vi "radio_set_generate_msg.vi"(8 "error in":errorcluster, 9 "Radio command":u16(ring) items=["op mode", "frequency", "power", "spread factor", "freq correction", "RX signal bw", "bitrate", "freq deviation", "preamble length", "crc", "bandwidth"], 10 "input parameter":string, 11 "VISA in":refnum<visa-resource-name>) -> (0 "error out":errorcluster, 1 "error":bool, 2 "output command":string, 3 "VISA out":refnum<visa-resource-name>)   [LabVIEW 2011]
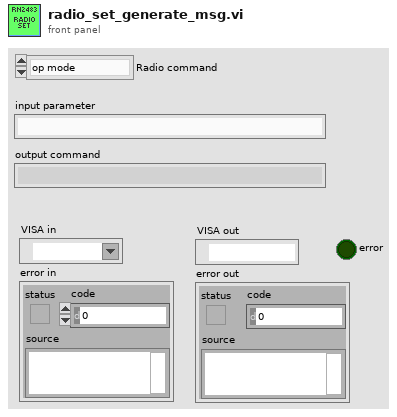
[diagram p1: front panel]
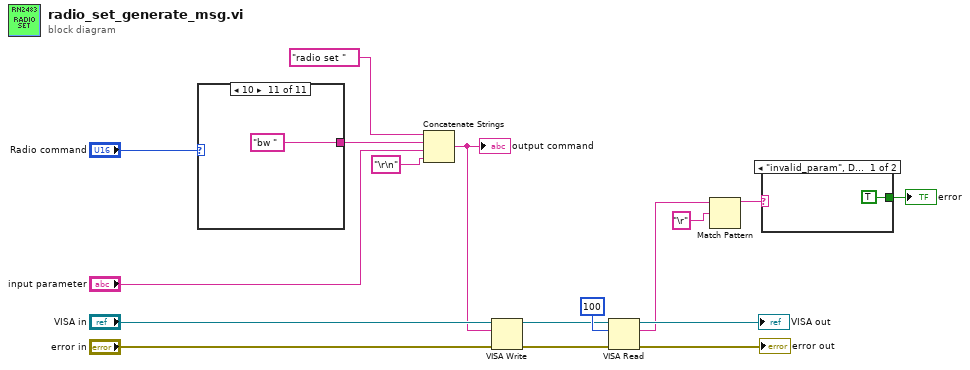
[diagram p0: block diagram]
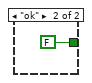
[diagram p2: hidden frame]
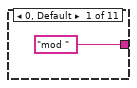
[diagram p3: hidden frame]
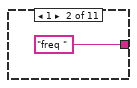
[diagram p4: hidden frame]
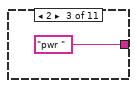
[diagram p5: hidden frame]
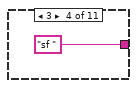
[diagram p6: hidden frame]
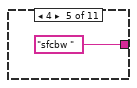
[diagram p7: hidden frame]
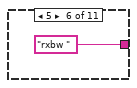
[diagram p8: hidden frame]
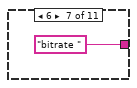
[diagram p9: hidden frame]
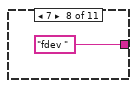
[diagram p10: hidden frame]
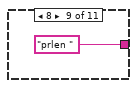
[diagram p11: hidden frame]
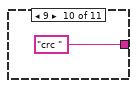
[diagram p12: hidden frame]
diagram:
  n1 = case shown="10" "Radio command" {
    tunnel: ["mod " "freq " "pwr " "sf " "sfcbw " "rxbw " "bitrate " "fdev " "prlen " "crc " "bw "] -> w15
    frame 0, Default {
    }
    frame 1 {
    }
    frame 2 {
    }
    frame 3 {
    }
    frame 4 {
    }
    frame 5 {
    }
    frame 6 {
    }
    frame 7 {
    }
    frame 8 {
    }
    frame 9 {
    }
    frame 10 {
    }
  }
  n2 = Concatenate Strings("radio set ", w15, "input parameter", "\r\n") -> (w7:string)
  "output command" <- w7
  n3 = VISA Write(VISA resource name="VISA in", write buffer=w7, error in (no error)="error in") -> (VISA resource name out=w9:refnum<visa-resource-name>, error out=w8:errorcluster)  [unwired: 1 out]
  n4 = VISA Read(VISA resource name=w9, byte count=u32 100, error in (no error)=w8) -> (VISA resource name out=→"VISA out":refnum<visa-resource-name>, read buffer=w3:string, error out=→"error out":errorcluster)  [unwired: 1 out]
  n5 = Match Pattern(string=w3, regular expression="\r" ("string to write")) -> (before substring=w2:string)  [unwired: 1 in, 3 out]
  n6 = case shown="\"invalid_param\", Default" w2 {
    tunnel: [TRUE FALSE] -> w1
    frame "invalid_param", Default {
    }
    frame "ok" {
    }
  }
  "error" <- w1
